vi "draw_track7_image_diplay.vi"(2 "GOALpos":cluster{"X":sgl, "Y":sgl}[](array[cluster])=[{"X"=630.0, "Y"=680.0}, {"X"=67.0, "Y"=153.0}, {"X"=74.0, "Y"=630.0}], 3 "角度阈值":dbl=60.0 format="%#_13g", 4 "距离阈值":dbl=1000.0 format="%#_13g", 5 "bin_billard":T1, 6 "color_billard":T1) -> (0 "color_billard 2":T1, 1 "大小":i32)   [LabVIEW 2018]
uses:
  <vilib>/vision/Shape Detection.llb/ShapeDetectionMatchOptions.ctl
  <vilib>/vision/Pattern Matching.llb/IMAQ Match Range Setting.ctl
  <vilib>/vision/Image Controls.llb/IMAQ Image.ctl
  <vilib>/vision/NI_Vision_Development_Module.lvlib
panel:
  out "Image":T1(plugin-control)
  in  "color":path
  in  "Match Options":T2={"Rotation"=TRUE, "Scale"=FALSE, "Occlusion"=FALSE, "Range Settings"=[]} {"Range Settings"."Match Constraints" items=["Rotation Angle (degrees)", "Scale Factor (%)", "Occlusion (%)"]}
  out "endX":dbl format="%#_13g"
  out "endY":dbl format="%#_13g"
  # "Range"
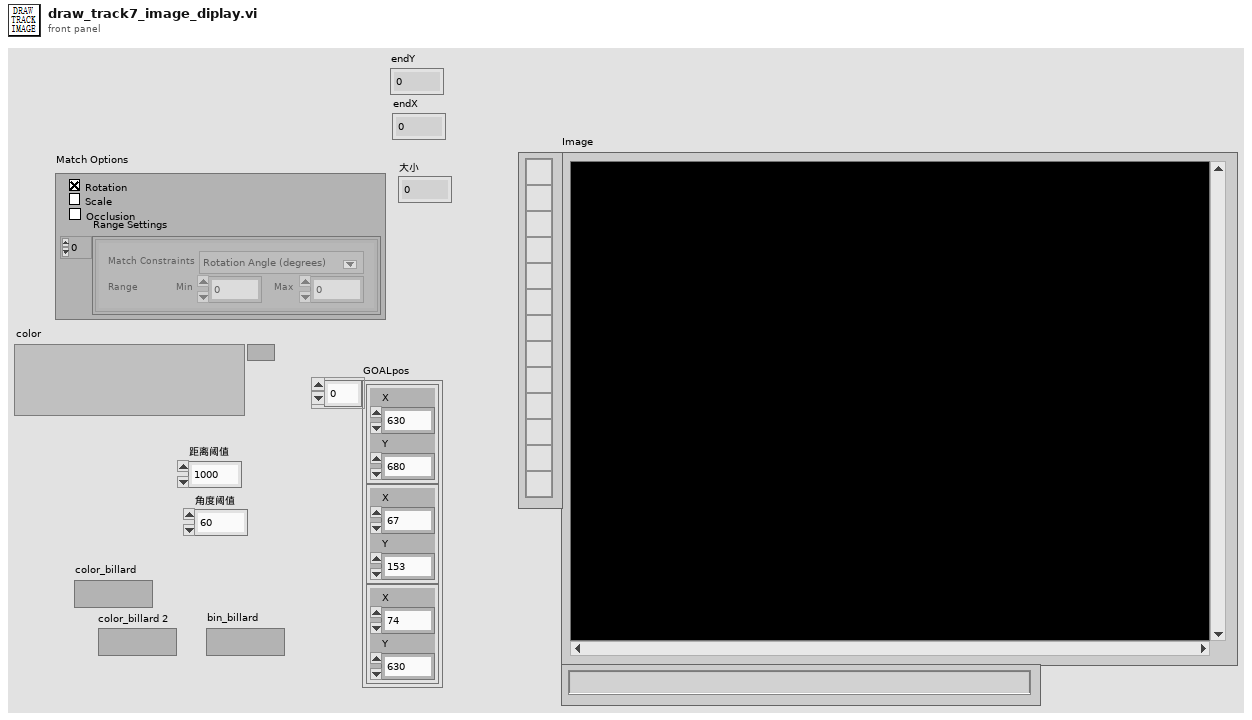
[diagram p1: front panel]
types:
  T1 = typedef "IMAQ Image.ctl" = refnum<image>
  T2 = typedef "ShapeDetectionMatchOptions.ctl" = cluster{"Rotation":bool, "Scale":bool, "Occlusion":bool, "Range Settings":T3[]}
  T3 = typedef "IMAQ Match Range Setting.ctl" = cluster{"Match Constraints":u32, "Min":dbl, "Max":dbl}
  T4 = cluster{"Position":cluster{"X":sgl, "Y":sgl}, "Radius":dbl, "Score":dbl}[]
  T5 = cluster{"Position":cluster{"X":sgl, "Y":sgl}, "Radius":dbl, "Score":dbl}
  T6 = cluster{i32, i32, "X Resolution":i32, "Y Resolution":i32}
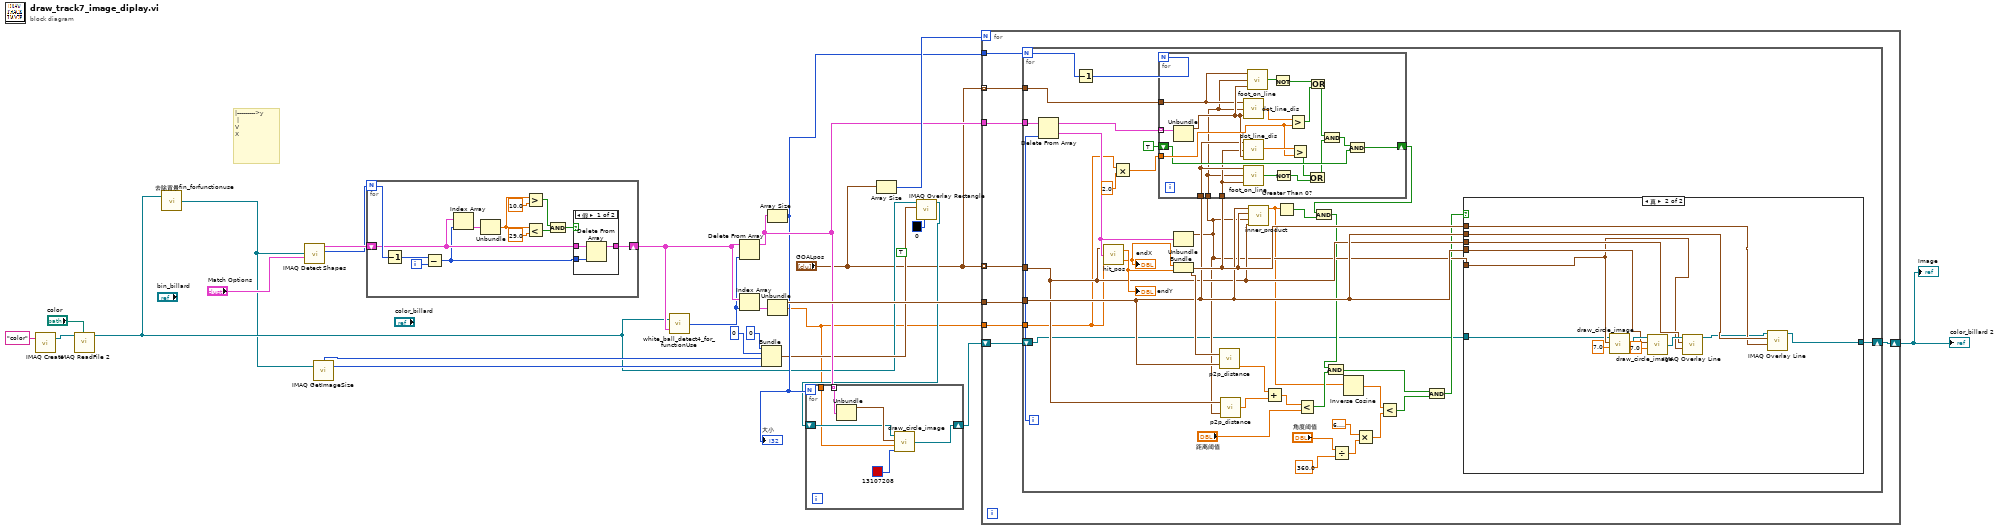
[diagram p0: block diagram]
diagram:
  (unwired) TRUE ("fill?(F)")
  # "|--------->y\n |\nV\nX"
  n1 = call "IMAQ Create"("Image Name"="color") -> ("New Image"=w8:T1)  [unwired: 4 in, 1 out]
  n2 = call "IMAQ ReadFile 2"("File Path"="color", "Image"=w8) -> ("Image Out"=w4:T1)  [unwired: 5 in, 4 out]
  n3 = call "去除背景fin_forfunctionuse.vi"("Image Src"=w4) -> ("Image Out"=w3:T1)  [unwired: 1 in]
  n4 = call-poly "IMAQ Detect Shapes"("Match Options"="Match Options", "Image"=w3) -> ("Number of Matches Returned"=w24:i32, "Circles"=w25:T4)  [unwired: 7 in, 1 out]
  n5 = call "IMAQ GetImageSize"("Image"=w3) -> ("Y Resolution"=w16:i32, "X Resolution"=w15:i32)  [unwired: 3 in, 1 out]
  n6 = for {
    N: w24 -> [w34]
    shift-right: [w28] -> w20
    shift-left: w25 -> [w29]
    i -> [w32]
    n7 = Decrement(x=w34) -> (x-1=w33:i32)
    n8 = Subtract(x=w33, y=w32) -> (x-y=w27:i32)
    n9 = Index Array(array=w29, index=w27) -> (element=w31:T5)
    n10 = Unbundle(w31) -> ("Radius"=w38:dbl)  [unwired: 2 out]
    n11 = Greater?(x=w38, y=10.0) -> (0:w36:bool)
    n12 = Less?(x=w38, y=29.0) -> (x < y?=w35:bool)
    n13 = And(x=w36, y=w35) -> (x .and. y?=w30:bool)
    n14 = case shown="假" w30 {
      tunnel: w29 -> [w42 w43]
      tunnel: [w41 w43] -> w28
      tunnel: w27 -> [w40 _]
      frame False {
        n15 = Delete From Array(array=w42, index=w40) -> (array with subset deleted=w41:T4)  [unwired: 1 in, 1 out]
      }
      frame True {
      }
    }
  }
  n16 = call "white_ball_detect4_for_functionUse.vi"("Circles"=w20, "color_billard"=w4) -> ("白球所在(已处理的)数组位置"=w19:i32)
  n17 = Delete From Array(array=w20, index=w19) -> (array with subset deleted=w14:T4)  [unwired: 1 in, 1 out]
  n18 = Index Array(array=w20, index=w19) -> (element=w23:T5)
  n19 = Bundle(0, 0, "X Resolution"=w15, "Y Resolution"=w16) -> (w12:T6)  [unwired: 1 in]
  n20 = Array Size(array=w14) -> (size(s)=w13:i32)
  "大小" <- w13
  n21 = Unbundle(w23) -> ("Position"=w22:cluster{"X":sgl, "Y":sgl}, "Radius"=w1:dbl)  [unwired: 1 out]
  n22 = Array Size(array="GOALpos") -> (size(s)=w21:i32)
  n23 = call "IMAQ Overlay Rectangle"("Color"=u32 0, "Rectangle"=w12, "Image"=w4) -> ("Image Out"=w10:T1)  [unwired: 7 in, 1 out]
  n24 = for {
    N: w13 -> [_]
    tunnel: w14 -> [w49] mode=indexing
    shift-right: [w46] -> w9
    shift-left: w10 -> [w47]
    tunnel: w1 -> [w44]
    n25 = Unbundle(w49) -> ("Position"=w48:cluster{"X":sgl, "Y":sgl})  [unwired: 2 out]
    n26 = call "draw_circle_image.vi"("Color"=u32 13107208, "radius"=w44, "Position"=w48, "Image"=w47) -> ("Image Out"=w46:T1)
  }
  n27 = for {
    N: w21 -> [_]
    tunnel: w22 -> [w57]
    tunnel: w13 -> [w56]
    tunnel: "GOALpos" -> [w55] mode=indexing
    tunnel: w14 -> [w54]
    tunnel: w1 -> [w53]
    shift-right: [w52] -> w5
    shift-left: w9 -> [w51]
    tunnel: "GOALpos" -> [w50] mode=indexing
    n28 = for {
      N: w56 -> [w92]
      tunnel: w57 -> [w82]
      tunnel: w55 -> [w81]
      tunnel: w54 -> [w86]
      tunnel: w53 -> [w61]
      shift-right: [w63] -> w52
      shift-left: w51 -> [w62]
      tunnel: w50 -> [w58]
      i -> [w87]
      n29 = Delete From Array(array=w86, index=w87) -> (deleted portion=w85:T5, array with subset deleted=w90:T4)  [unwired: 1 in]
      n30 = Decrement(x=w92) -> (x-1=w91:i32)
      n31 = call "hit_pos.vi"("radius"=w61, "TARGET Circle Descriptor"=w85, "GOALpos"=w81) -> ("endX"=w93:dbl, "endY"=w94:dbl)
      "endY" <- w94
      "endX" <- w93
      n32 = Multiply(x=w61, y=2.0) -> (x*y=w59:dbl)
      n33 = Unbundle(w85) -> ("Position"=w80:cluster{"X":sgl, "Y":sgl})  [unwired: 2 out]
      n34 = Bundle("endX"=w93, "endY"=w94) -> (w83:cluster{"endX":dbl, "endY":dbl})  [unwired: 1 in]
      n35 = for {
        N: w91 -> [_]
        tunnel: w58 -> [w106]
        tunnel: w90 -> [w114] mode=indexing
        tunnel: w80 -> [w97]
        tunnel: w82 -> [w104]
        tunnel: w83 -> [w103]
        tunnel: w59 -> [w111]
        shift-right: [w108] -> w84
        shift-left: TRUE -> [w109]
        n36 = Unbundle(w114) -> ("Position"=w107:cluster{"X":sgl, "Y":sgl})  [unwired: 2 out]
        n37 = call "dot_line_dis.vi"("dot pos"=w107, "line end"=w97, "line start"=w106) -> ("distance"=w113:sgl)
        n38 = call "dot_line_dis.vi"("dot pos"=w107, "line end"=w103, "line start"=w104) -> ("distance"=w112:sgl)
        n39 = call "foot_on_line.vi"("dot"=w103, "line end"=w97, "line start"=w104) -> ("foot on line？"=w101:bool)
        n40 = call "foot_on_line.vi"("dot"=w107, "line end"=w97, "line start"=w106) -> ("foot on line？"=w102:bool)
        n41 = Not(x=w102) -> (.not. x?=w96:bool)
        n42 = Not(x=w101) -> (.not. x?=w95:bool)
        n43 = Greater?(x=w113, y=w111) -> (0:w105:bool)
        n44 = Greater?(x=w112, y=w111) -> (0:w100:bool)
        n45 = Or(x=w100, y=w95) -> (x .or. y?=w98:bool)
        n46 = Or(x=w96, y=w105) -> (x .or. y?=w99:bool)
        n47 = And(x=w99, y=w98) -> (x .and. y?=w110:bool)
        n48 = And(x=w110, y=w109) -> (x .and. y?=w108:bool)
      }
      n49 = call "p2p_distance.vi"("point2"=w82, "point1"=w83) -> ("poit2poit_dis"=w79:dbl)
      n50 = call "p2p_distance.vi"("point2"=w80, "point1"=w81) -> ("poit2poit_dis"=w78:dbl)
      n51 = call "inner_product.vi"("L2ENDpos"=w81, "L2STARTpos"=w80, "L1ENDpos"=w83, "L1STARTpos"=w82) -> ("数值"=w73:dbl)  [unwired: 7 in]
      n52 = Add(x=w79, y=w78) -> (x+y=w77:dbl)
      n53 = Greater Than 0?(x=w73) -> (x > 0?=w89:bool)
      n54 = Less?(x=w77, y="距离阈值") -> (x < y?=w74:bool)
      n55 = And(x=w84, y=w89) -> (x .and. y?=w75:bool)
      n56 = And(x=w75, y=w74) -> (x .and. y?=w70:bool)
      n57 = Divide(x="角度阈值", y=360.0) -> (x/y=w66:dbl)
      n58 = Inverse Cosine(1:w73) -> (0:w72:dbl)
      n59 = Multiply(x=6.283185307179586, y=w66) -> (x*y=w67:dbl)
      n60 = Less?(x=w72, y=w67) -> (x < y?=w71:bool)
      n61 = And(x=w70, y=w71) -> (x .and. y?=w69:bool)
      n62 = case shown="真" w69 {
        tunnel: w81 -> [_ w124]
        tunnel: w80 -> [_ w123]
        tunnel: w82 -> [_ w122]
        tunnel: w83 -> [_ w121]
        tunnel: w82 -> [_ w126]
        tunnel: [w115 w119] -> w63
        tunnel: w62 -> [w115 w116]
        frame False {
        }
        frame True {
          n63 = call "draw_circle_image.vi"("radius"=7.0, "Position"=w123, "Image"=w116) -> ("Image Out"=w127:T1)  [unwired: 1 in]
          n64 = call "draw_circle_image.vi"("radius"=7.0, "Position"=w126, "Image"=w127) -> ("Image Out"=w125:T1)  [unwired: 1 in]
          n65 = call "IMAQ Overlay Line"("End Point"=w123, "Start Point"=w124, "Image"=w125) -> ("Image Out"=w120:T1)  [unwired: 7 in, 1 out]
          n66 = call "IMAQ Overlay Line"("End Point"=w121, "Start Point"=w122, "Image"=w120) -> ("Image Out"=w119:T1)  [unwired: 7 in, 1 out]
        }
      }
    }
  }
  "color_billard 2" <- w5
  "Image" <- w5
